vi "CS-4 Get Operational Mode.vi"(0 "VISA session":refnum<visa-resource-name>, 2 "error in (no error)":errorcluster) -> (3 "dup VISA session":refnum<visa-resource-name>, 4 "response out":string, 5 "Mode":enum16{"Manual", "Auto"}(ring), 6 "error out":errorcluster)   [LabVIEW 2020]
doc: "CS-4 Get Operational Mode.vi will return the operating mode (manual or auto)."
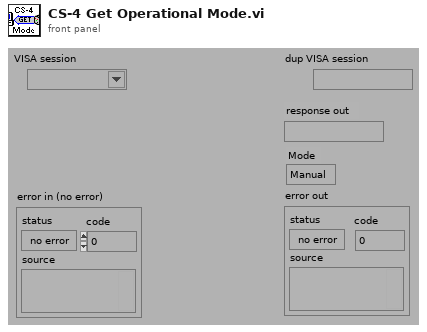
[diagram p1: front panel]
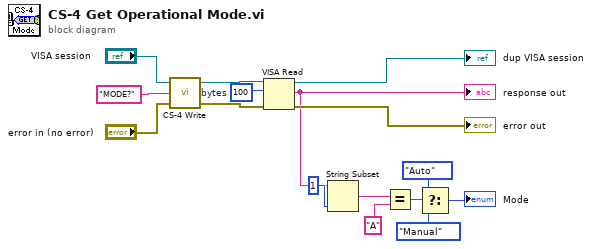
[diagram p0: block diagram]
diagram:
  w12 = u32 100  # bytes
  n1 = call "CS-4 Write.vi"("error in (no error)"="error in (no error)", "write buffer (\"\")"="MODE?", "VISA session"="VISA session") -> ("error out"=w13:errorcluster, "dup VISA session"=w14:refnum<visa-resource-name>)  [unwired: 1 out]
  n2 = VISA Read(VISA resource name=w14, byte count=w12, error in (no error)=w13) -> (VISA resource name out=→"dup VISA session":refnum<visa-resource-name>, read buffer=w5:string, error out=→"error out":errorcluster)  [unwired: 1 out]
  "response out" <- w5
  n3 = String Subset(string=w5, length (rest)=1 ("length")) -> (substring=w7:string)  [unwired: 1 in]
  n4 = Equal?(x=w7, y="A") -> (x = y?=w4:bool)
  n5 = Select(t=enum16{"Manual", "Auto"}."Auto" ("units"), s=w4, f=enum16{"Manual", "Auto"}."Manual" ("units")) -> (s? t:f=→"Mode":enum16{"Manual", "Auto"})
